vi "StartProcess.vi"(0 "reference in":refnum<class "Tester.lvclass">, 3 "ms timeout (-1)":i32=-1, 5 "error in (no error)":errorcluster) -> (14 "reference out":refnum<class "Tester.lvclass">, 15 "EventFromProcess":refnum<user-event>, 16 "timed out":bool, 18 "ProcessViRef":refnum<vi>, 19 "error out":errorcluster)   [LabVIEW 2020, in "Tester.lvclass"]
doc: "Looks up an existing object matching object name or creates a new object and returns a refnum you can use when calling other class methods.\n\nObjects created with this VI should be destroyed using this class Delete VI."
uses:
  Tester.lvclass
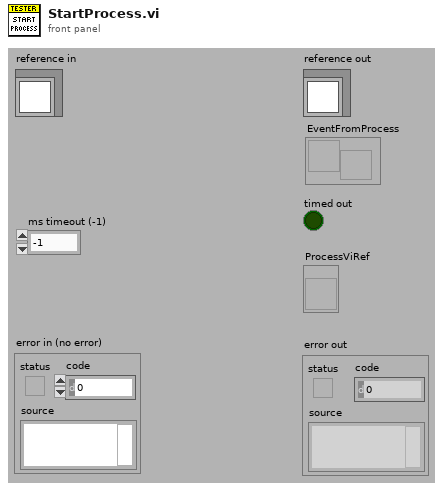
[diagram p1: front panel]
types:
  T1 = enum16{"ReadRepository", "CreateNew", "CreateOrLookUpExisting", "ReadRepositoryAndDestroy"}
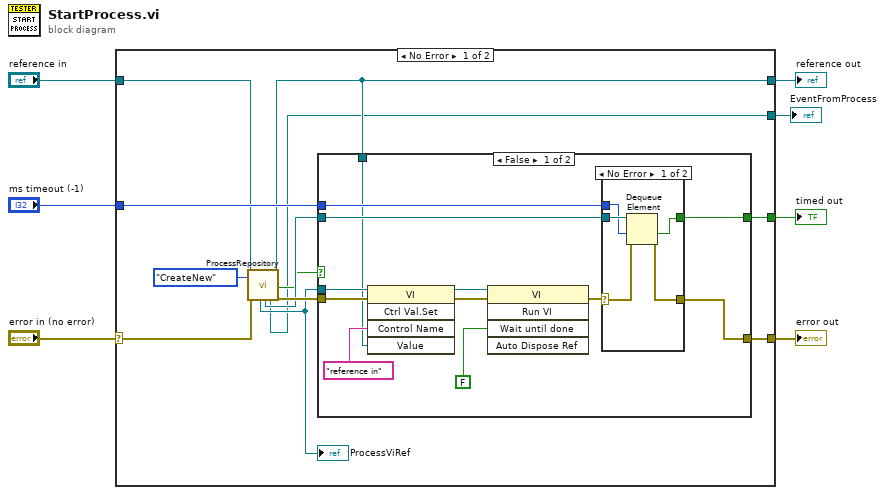
[diagram p0: block diagram]
diagram:
  n1 = case shown="No Error" "error in (no error)" {
    selector: "error in (no error)" -> [w16 w39]
    tunnel: [w17 w39] -> w6
    tunnel: [w12 w40] -> w4
    tunnel: "reference in" -> [w10 w40]
    tunnel: "ms timeout (-1)" -> [w19 _]
    tunnel: [w18 _] -> w2
    tunnel: [w9 _] -> w1
    frame No Error {
      n2 = call "ProcessRepository.vi"("reference in"=w10, "Action(ReadRepository)"=T1."CreateNew", "error in (no error)"=w16) -> ("ProcessViRef"=w14:refnum<vi>, "ProcessSyncQueue"=w13:refnum<queue>, "EventFromProcess"=w9:refnum<user-event>, "reference out"=w12:refnum<class "Tester.lvclass">, "ProcessAlreadyStarted"=w11:bool, "error out"=w15:errorcluster)  [unwired: 9 in, 2 out]
      "ProcessViRef" <- w14
      n3 = case shown="False" w11 {
        tunnel: w19 -> [w27 _]
        tunnel: [w26 _] -> w18
        tunnel: [w24 w38] -> w17
        tunnel: w15 -> [w23 w38]
        tunnel: w14 -> [w22 _]
        tunnel: w13 -> [w21 _]
        tunnel: w12 -> [w20 _]
        frame False {
          n4 = invoke class="VI" method="Ctrl Val.Set"(reference=w22, error in=w23, "Control Name"="reference in", "Value"=w20) -> (reference out=w30:refnum<vi>, error out=w29:errorcluster)  [unwired: 1 in, 3 out]
          n5 = invoke class="VI" method="Run VI"(reference=w30, error in=w29, "Wait until done"=FALSE ("Wait Until Done")) -> (error out=w25:errorcluster)  [unwired: 2 in, 4 out]
          n6 = case shown="No Error" w25 {
            tunnel: w21 -> [w36 _]
            tunnel: w27 -> [w34 _]
            tunnel: [w35 _] -> w26
            selector: w25 -> [w33 w37]
            tunnel: [w32 w37] -> w24
            frame No Error {
              n7 = Dequeue Element(queue=w36, timeout in ms (-1)=w34, error in (no error)=w33) -> (timed out?=w35:bool, error out=w32:errorcluster)  [unwired: 2 out]
            }
            frame Error {
            }
          }
        }
        frame True {
          # "Process Already started.\nThis option will only be used togeather with the\naction: \"CreateOrLookUpExisting\""
        }
      }
    }
    frame Error {
    }
  }
  "error out" <- w6
  "reference out" <- w4
  "timed out" <- w2
  "EventFromProcess" <- w1
